vi "CTRE_Tank_Servo_Straight_Imu.vi"(6 "Servo Params":T10, 7 "PigeonIMU":T7={"DeviceStatus"={"status"=FALSE, "code"=0, "source"=""}, "Device Number"=0, "Type"=352321536, "Device ID"=0, "Handle"=0, "UsageFrame"=0, "Library Path"=path ""} {"Type" items=["CAN"=352321536, "TalonSRX"=33554432]}, 8 "Forward":dbl format="%#_13g", 9 "Set Heading":dbl, 10 "Talon SRX Control Mode":T9, 11 "Tank Drivetrain":T1) -> (0 "Heading Good":bool, 2 "Tank Straight IMU":T11 {"PigeonIMU"."Type" items=["CAN"=352321536, "TalonSRX"=33554432]}, 3 "Tank Drivetrain":T1={"Left Gearbox"={"SmartMotorController 1"={"DeviceStatus"={"status"=FALSE, "code"=0, "source"=""}, "Type"=enum."PWM", "PWM"={"PWM Channel"=enum."PWM 1", "DeadBand"={"Name"="", "maxPositivePwm"=0, "minPositivePwm"=0, "centerPwm"=0, "maxNegativePwm"=0, "minNegativePwm"=0, "angularRange"=0}}, "CAN"={"Device Number"=0, "SetOutput VI Ref"=variant(enum8{"Percent VBus", "Current", "Speed", "Position", "Voltage"} enum."Percent VBus"), "GetOutput VI Ref"=variant(refnum<k1> refnum), "Enable VI Ref"=variant(dbl 12.0), "Disable VI Ref"=variant(enum8{"Percent VBus", "Speed", "Position", "Slave", "Unchanged / Invalid", "Voltage Compensation", "Current", "Motion Profile"} enum."Percent VBus"), "Data"=variant}, "Invert"=FALSE}, "Invert"=FALSE}, "Right Gearbox"={"SmartMotorController 1"={"DeviceStatus"={"status"=FALSE, "code"=0, "source"=""}, "Type"=enum."PWM", "PWM"={"PWM Channel"=enum."PWM 1", "DeadBand"={"Name"="", "maxPositivePwm"=0, "minPositivePwm"=0, "centerPwm"=0, "maxNegativePwm"=0, "minNegativePwm"=0, "angularRange"=0}}, "CAN"={"Device Number"=0, "SetOutput VI Ref"=variant(enum8{"Percent VBus", "Current", "Speed", "Position", "Voltage"} enum."Percent VBus"), "GetOutput VI Ref"=variant(refnum<k1> refnum), "Enable VI Ref"=variant(dbl 12.0), "Disable VI Ref"=variant(enum8{"Percent VBus", "Speed", "Position", "Slave", "Unchanged / Invalid", "Voltage Compensation", "Current", "Motion Profile"} enum."Percent VBus"), "Data"=variant}, "Invert"=FALSE}, "Invert"=FALSE}})   [LabVIEW 2016]
uses:
  <vilib>/Rock Robotics/WPI/ThirdParty/CanMotor/CTRLib-LV-TalonSRX/Framework/Tank.ctl
  <vilib>/Rock Robotics/WPI/ThirdParty/CanMotor/CTRLib-LV-TalonSRX/Framework/Gearbox.ctl
  <vilib>/Rock Robotics/WPI/MotorControl/WPI_MotorControlDeviceRef.ctl
  <vilib>/Rock Robotics/WPI/MotorControl/WPI_MotorControlType.ctl
  <vilib>/Rock Robotics/SystemInterfaces/DIO/FPGA_DIOPWMChannel.ctl
  <vilib>/Rock Robotics/WPI/PWM/WPI_PWMDeadband.ctl
  <vilib>/Rock Robotics/WPI/ThirdParty/Sensors/Pigeon IMU/CTRE_PigeonIMU_DeviceRef.ctl
  <vilib>/Rock Robotics/WPI/ThirdParty/Sensors/Pigeon IMU/CTRE_PigeonIMU_ConnectionType.ctl
  <vilib>/Rock Robotics/WPI/ThirdParty/CanMotor/CTRLib-LV-TalonSRX/CTRE_CANTalonSRX_ControlMode.ctl
  <vilib>/Rock Robotics/WPI/ThirdParty/CanMotor/CTRLib-LV-TalonSRX/Framework/ServoParams.ctl
  <vilib>/Rock Robotics/WPI/ThirdParty/Sensors/Pigeon IMU/CTRE_PigeonIMU_GetRawGyro.vi
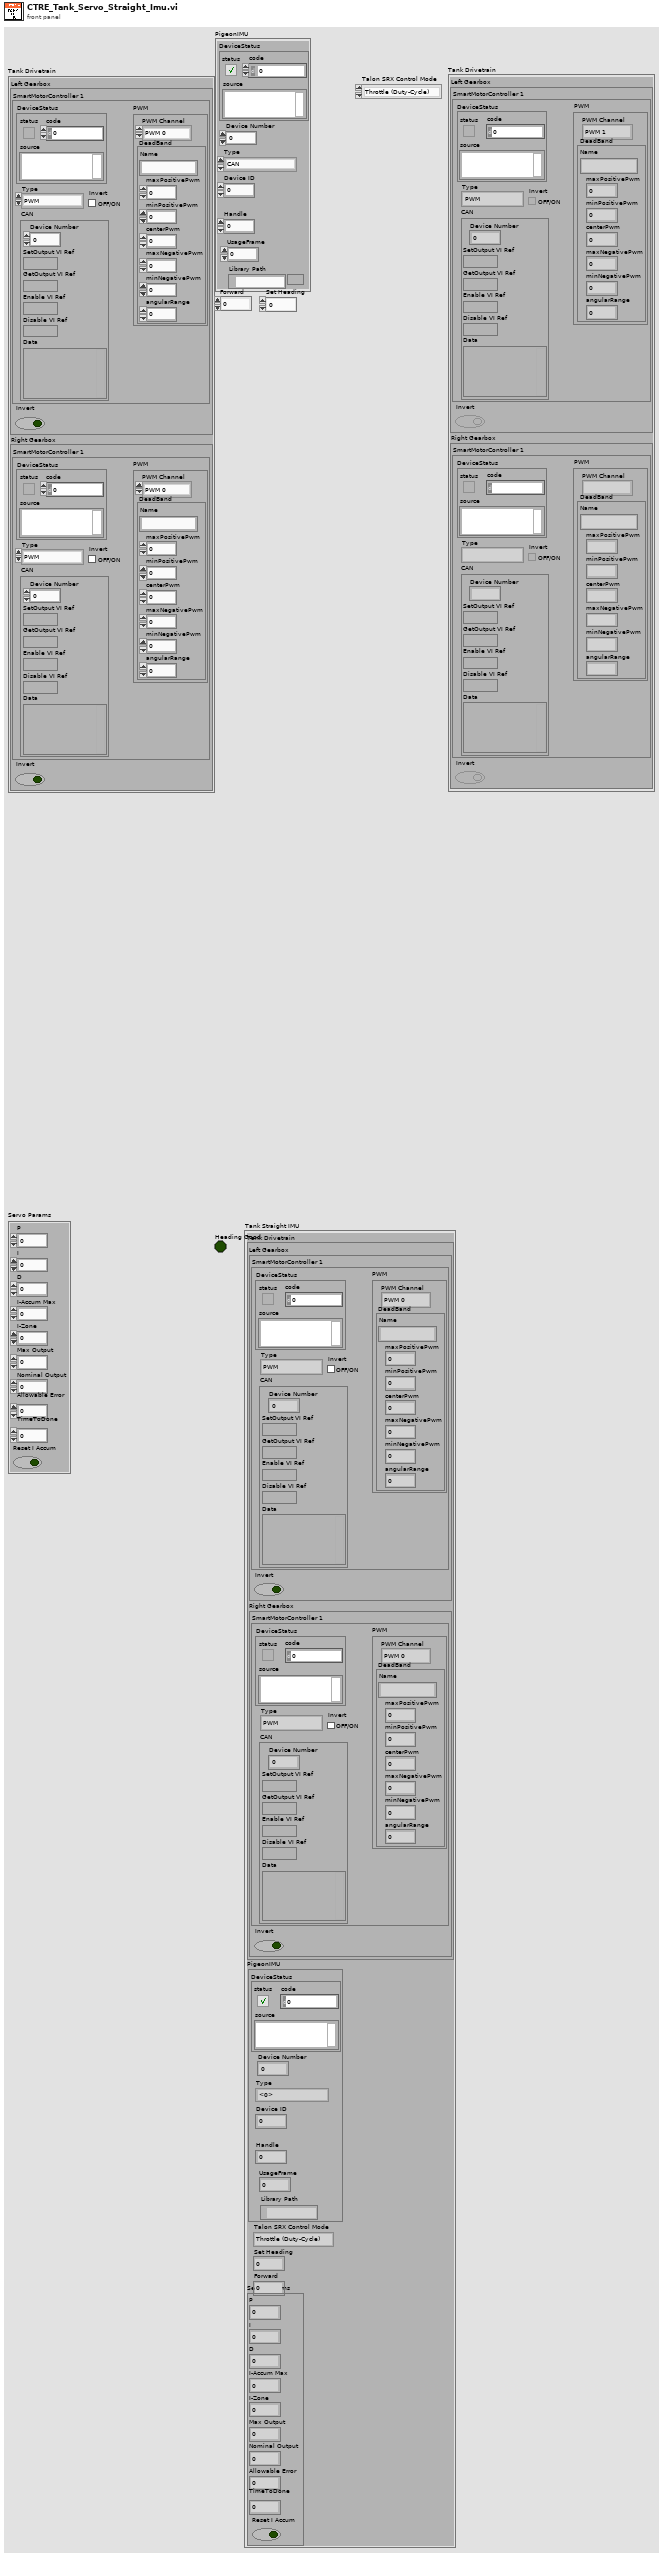
[diagram p1: front panel]
types:
  T1 = typedef "Tank.ctl" = cluster{"Left Gearbox":T2, "Right Gearbox":T2}
  T2 = typedef "Gearbox.ctl" = cluster{"SmartMotorController 1":T3, "Invert":bool}
  T3 = typedef "WPI_MotorControlDeviceRef.ctl" = cluster{"DeviceStatus":errorcluster, "Type":T4, "PWM":cluster{"PWM Channel":T5, "DeadBand":T6}, "CAN":cluster{"Device Number":u8, "SetOutput VI Ref":variant, "GetOutput VI Ref":variant, "Enable VI Ref":variant, "Disable VI Ref":variant, "Data":variant}, "Invert":bool}
  T4 = typedef "WPI_MotorControlType.ctl" = enum16{"PWM", "CAN"}
  T5 = typedef "FPGA_DIOPWMChannel.ctl" = enum8{"PWM 0", "PWM 1", "PWM 2", "PWM 3", "PWM 4", "PWM 5", "PWM 6", "PWM 7", "PWM 8", "PWM 9", "PWM MXP 0", "PWM MXP 1", "PWM MXP 2", "PWM MXP 3", "PWM MXP 4", "PWM MXP 5", "PWM MXP 6", "PWM MXP 7", "PWM MXP 8", "PWM MXP 9", "Invalid"}
  T6 = typedef "WPI_PWMDeadband.ctl" = cluster{"Name":string, "maxPositivePwm":i32, "minPositivePwm":i32, "centerPwm":i32, "maxNegativePwm":i32, "minNegativePwm":i32, "angularRange":u16}
  T7 = typedef "CTRE_PigeonIMU_DeviceRef.ctl" = cluster{"DeviceStatus":errorcluster, "Device Number":u8, "Type":T8, "Device ID":u32, "Handle":u64, "UsageFrame":u32, "Library Path":path}
  T8 = typedef "CTRE_PigeonIMU_ConnectionType.ctl" = u32
  T9 = typedef "CTRE_CANTalonSRX_ControlMode.ctl" = enum16{"Throttle (Duty-Cycle)", "Position Closed-Loop", "Velocity Closed-Loop", "Current Closed-Loop", "Voltage Compensation", "Slave Follower", "Motion Profile", "Motion Magic"}
  T10 = typedef "ServoParams.ctl" = cluster{"P":dbl, "I":dbl, "D":dbl, "I-Accum Max":dbl, "I-Zone":dbl, "Max Output":dbl, "Nominal Output":dbl, "Allowable Error":dbl, "TimeToDone":dbl, "Reset I Accum":bool}
  T11 = cluster{"Tank Drivetrain":T1, "PigeonIMU":T7, "Talon SRX Control Mode":T9, "Set Heading":dbl, "Forward":dbl, "Servo Params":T10}
  T12 = cluster{"X":dbl, "Y":dbl, "Z":dbl, "Magnitude":dbl}
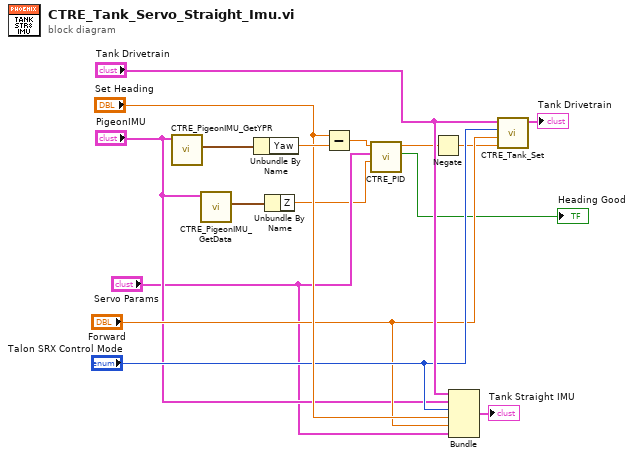
[diagram p0: block diagram]
diagram:
  n1 = call <vilib>:"CTRE_PigeonIMU_GetYPR.vi"("PigeonIMUDevRef"="PigeonIMU") -> ("Yaw Pitch Roll"=w13:cluster{"Yaw":dbl, "Pitch":dbl, "Roll":dbl})  [unwired: 8 in, 2 out]
  n2 = call-poly <vilib>:"CTRE_PigeonIMU_GetData.vi"("PigeonIMUDevRef"="PigeonIMU") -> ("Gyro DPS"=w7:T12)  [unwired: 8 in, 2 out]
  n3 = Unbundle By Name(w13) -> ("Yaw"=w16:dbl)
  n4 = Unbundle By Name(w7) -> ("Z"=w4:dbl)
  n5 = Subtract(x="Set Heading", y=w16) -> (x-y=w15:dbl)
  n6 = call <vilib>:"CTRE_PID.vi"("Sensor Derivative"=w4, "Servo Params"="Servo Params", "Error"=w15) -> ("At Target"=→"Heading Good":bool, "Out"=w3:dbl)  [unwired: 7 in]
  n7 = Negate(x=w3) -> (-x=w6:dbl)
  n8 = Bundle("Tank Drivetrain"="Tank Drivetrain", "PigeonIMU"="PigeonIMU", "Talon SRX Control Mode"="Talon SRX Control Mode", "Set Heading"="Set Heading", "Forward"="Forward", "Servo Params"="Servo Params") -> (→"Tank Straight IMU":T11)  [unwired: 1 in]
  n9 = call <vilib>:"CTRE_Tank_Set.vi"("Turn"=w6, "Forward"="Forward", "Talon SRX Control Mode"="Talon SRX Control Mode", "Tank Drivetrain"="Tank Drivetrain") -> ("Tank Drivetrain"=→"Tank Drivetrain":T1)  [unwired: 6 in, 1 out]
